vi "getAdditionalDataFromXMLNative.vi"(8 "error in (no error)":errorcluster, 10 "eventXML":refnum<k20>, 11 "RampEvent in":refnum<class "RampEvent.lvclass">) -> (0 "error out":errorcluster, 2 "eventXML out":refnum<k20>, 3 "RampEvent out":refnum<class "RampEvent.lvclass">)   [LabVIEW 2011, in "Tools.lvlib" / "Scripting.lvlib" / "RampEvent.lvclass"]
uses:
  RampEvent.lvclass
  RampEvent.lvclass/RampEvent.ctl
  <vilib>/xml/Close Reference(Node).vi
  <vilib>/xml/NI_XML.lvlib
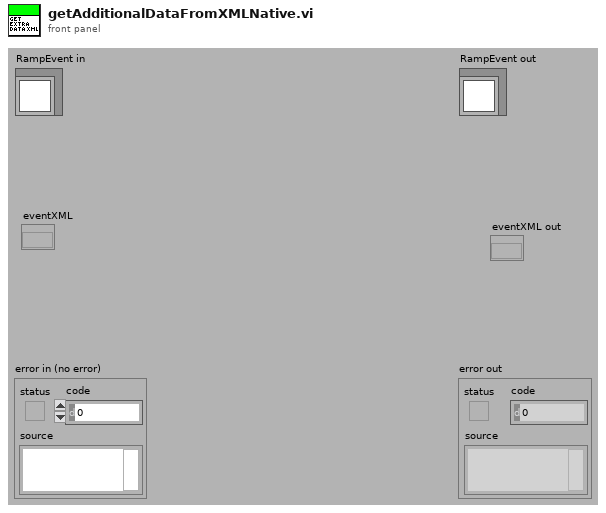
[diagram p1: front panel]
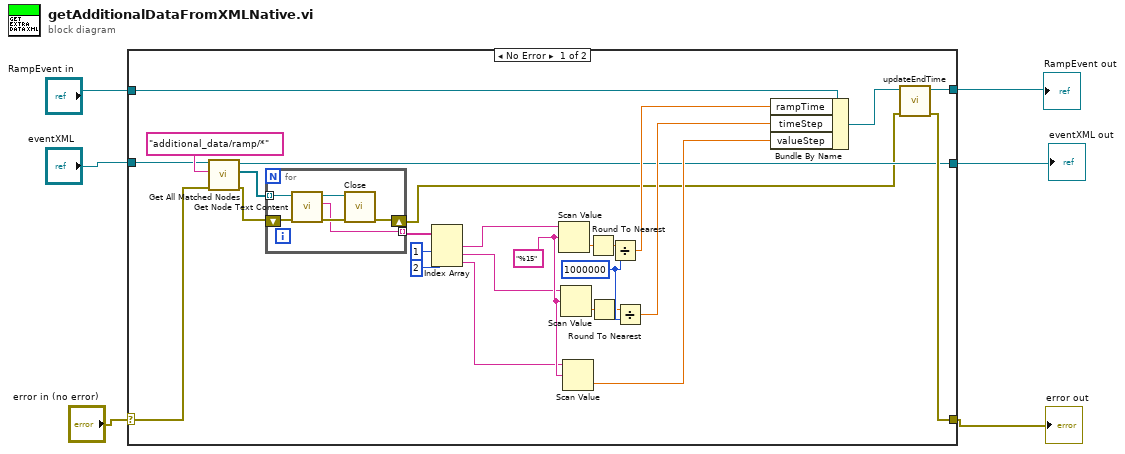
[diagram p0: block diagram]
diagram:
  n1 = case shown="No Error" "error in (no error)" {
    selector: "error in (no error)" -> [w15 w39]
    tunnel: [w22 w39] -> w3
    tunnel: "RampEvent in" -> [w27 w40]
    tunnel: [w23 w40] -> w4
    tunnel: "eventXML" -> [w16 _]
    tunnel: [w14 _] -> w1
    frame No Error {
      w30 = 1000000
      w26 = "%15"
      n2 = call <vilib>:"Get All Matched Nodes.vi"("error in (no error)"=w15, "XPath expression"="additional_data/ramp/*", "node in"=w16) -> ("error out"=w21:errorcluster, "node result array"=w19:refnum<k20>[], "node out"=w14:refnum<k20>)  [unwired: 6 in]
      n3 = for {
        tunnel: w19 -> [w35] mode=indexing
        tunnel: [w34] -> w18 mode=indexing
        shift-right: [w33] -> w9
        shift-left: w21 -> [w36]
        n4 = call <vilib>:"Get Node Text Content.vi"("error in (no error)"=w36, "node in"=w35) -> ("error out"=w37:errorcluster, "node text"=w34:string, "node out"=w38:refnum<k20>)  [unwired: 7 in]
        n5 = call-poly <vilib>:"Close.vi"("error in (no error)"=w37, "node"=w38) -> ("error out"=w33:errorcluster)  [unwired: 7 in]
      }
      n6 = Index Array(array=w18, index #2=1 ("index"), index #3=2 ("index")) -> (element #1=w12:string, element #2=w11:string, element #3=w10:string)  [unwired: 1 in]
      n7 = Scan Value(string=w12, format string=w26) -> (value=w32:dbl)  [unwired: 1 in, 1 out]
      n8 = Scan Value(string=w11, format string=w26) -> (value=w31:dbl)  [unwired: 1 in, 1 out]
      n9 = Scan Value(string=w10, format string=w26) -> (value=w25:dbl)  [unwired: 1 in, 1 out]
      n10 = Round To Nearest(number=w32) -> (nearest integer value=w8:dbl)
      n11 = Round To Nearest(number=w31) -> (nearest integer value=w7:dbl)
      n12 = Divide(x=w8, y=w30) -> (x/y=w29:dbl)
      n13 = Divide(x=w7, y=w30) -> (x/y=w28:dbl)
      n14 = Bundle By Name(cluster=w27, "rampTime"=w29, "timeStep"=w28, "valueStep"=w25) -> (w24:refnum<class "RampEvent.lvclass">)
      n15 = call-dynamic "updateEndTime.vi"("error in (no error)"=w9, "RampEvent in"=w24) -> ("error out"=w22:errorcluster, "RampEvent out"=w23:refnum<class "RampEvent.lvclass">)  [unwired: 8 in]
    }
    frame Error {
    }
  }
  "error out" <- w3
  "RampEvent out" <- w4
  "eventXML out" <- w1
